vi "DB Path.vi"() -> (0 "DB Path":string)   [LabVIEW 2015]
doc: "Returns the path to our database."
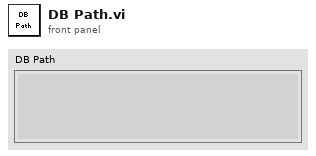
[diagram p1: front panel]
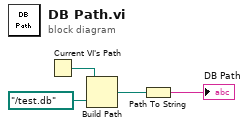
[diagram p0: block diagram]
diagram:
  n1 = Current VI's Path() -> (path=w4:path)
  n2 = Build Path(base path=w4, name or relative path=path "../test.db") -> (appended path=w2:path)
  n3 = Path To String(path=w2) -> (string=→"DB Path":string)
